vi "Do.vi"(8 "error in (no error)":errorcluster, 10 "Ctl Refnum in":refnum<vi>, 11 "ControlAction in":refnum<class "DoValueSignal.lvclass">) -> (0 "error out":errorcluster, 2 "Ctl Refnum out":refnum<vi>, 3 "ControlAction out":refnum<class "DoValueSignal.lvclass">)   [LabVIEW 2016, in "DoValueSignal.lvclass"]
uses:
  DoValueSignal.lvclass
  DoBase/ControlDoBase.lvclass
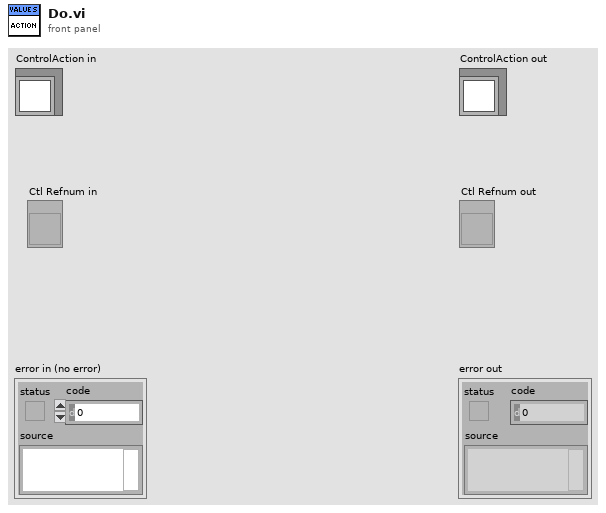
[diagram p1: front panel]
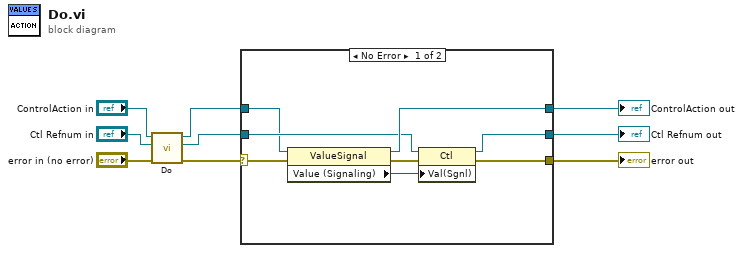
[diagram p0: block diagram]
diagram:
  n1 = call-parent "Do.vi"("error in (no error)"="error in (no error)", "Ctl Refnum in"="Ctl Refnum in", "ControlAction in"="ControlAction in") -> ("error out"=w3:errorcluster, "Ctl Refnum out"=w2:refnum<vi>, "ControlAction out"=w1:refnum<class "DoValueSignal.lvclass">)  [unwired: 6 in]
  n2 = case shown="No Error" w3 {
    selector: w3 -> [w14 w20]
    tunnel: [w17 w20] -> w6
    tunnel: [w16 w19] -> w5
    tunnel: [w15 w18] -> w4
    tunnel: w2 -> [w13 w19]
    tunnel: w1 -> [w11 w18]
    frame No Error {
      n3 = property class="ValueSignal"(reference=w11, error in=w14) -> (reference out=w15:refnum<class "DoValueSignal.lvclass">, error out=w12:errorcluster, "Value (Signaling)"=w10:variant)
      n4 = property class="Ctl"(reference=w13, error in=w12, "Val(Sgnl)"=w10) -> (reference out=w16:refnum<vi>, error out=w17:errorcluster)
    }
    frame Error {
    }
  }
  "error out" <- w6
  "ControlAction out" <- w4
  "Ctl Refnum out" <- w5
